vi "Main.vi"(8 "error in":errorcluster, 11 "SimulationDaq in":refnum<class "SimulationDaq.lvclass">) -> (0 "error out":errorcluster, 3 "SimulationDaq out":refnum<class "SimulationDaq.lvclass">)   [LabVIEW 2017, in "SimulationDaq.lvclass"]
doc: "The Queued Message Handler of a Worker."
uses:
  SimulationDaq.lvclass
  <vilib>/measure/NI_MABase.lvlib
  SDaqParameter.ctl
  <vilib>/addons/_Workers/Library/Classes/Message/Message.lvclass
  Initialization Data.ctl
  <vilib>/addons/_Workers/Library/Case Label.ctl
  <vilib>/addons/_Workers/Library/Workers.lvlib
  <vilib>/addons/_Workers/Library/Classes/Message Queue/Message Queue.lvclass
  <vilib>/addons/_Workers/Library/Classes/Message/Enqueue Message to Queue.vi
  <vilib>/addons/_Workers/Library/Classes/Worker/Worker.lvclass
  <vilib>/addons/_Workers/Library/Classes/Worker/Read ID.vi
  <vilib>/addons/_Workers/Library/Classes/Worker/Read Alias.vi
panel:
  out "ID out":string
  out "Alias out":string
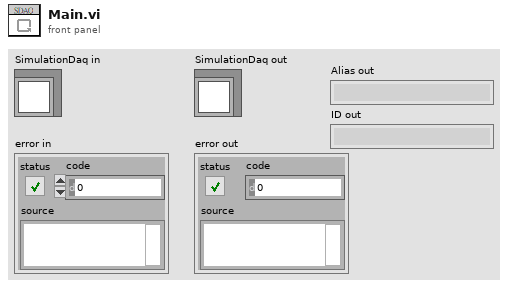
[diagram p1: front panel]
types:
  T1 = typedef "SimulationDaq.lvclass/Initialization Data.ctl" = cluster{"CallerEnQ":refnum<class "Message Queue.lvclass">, "ReturnCaseLabel":T2}
  T2 = typedef "Workers.lvlib/Case Label.ctl" = string
  T3 = typedef "SimulationDaq.lvclass/SDaqParameter.ctl" = cluster{"frequency":dbl, "amplitude":dbl, "sampling info":cluster{"Fs":dbl, "#s":dbl}}
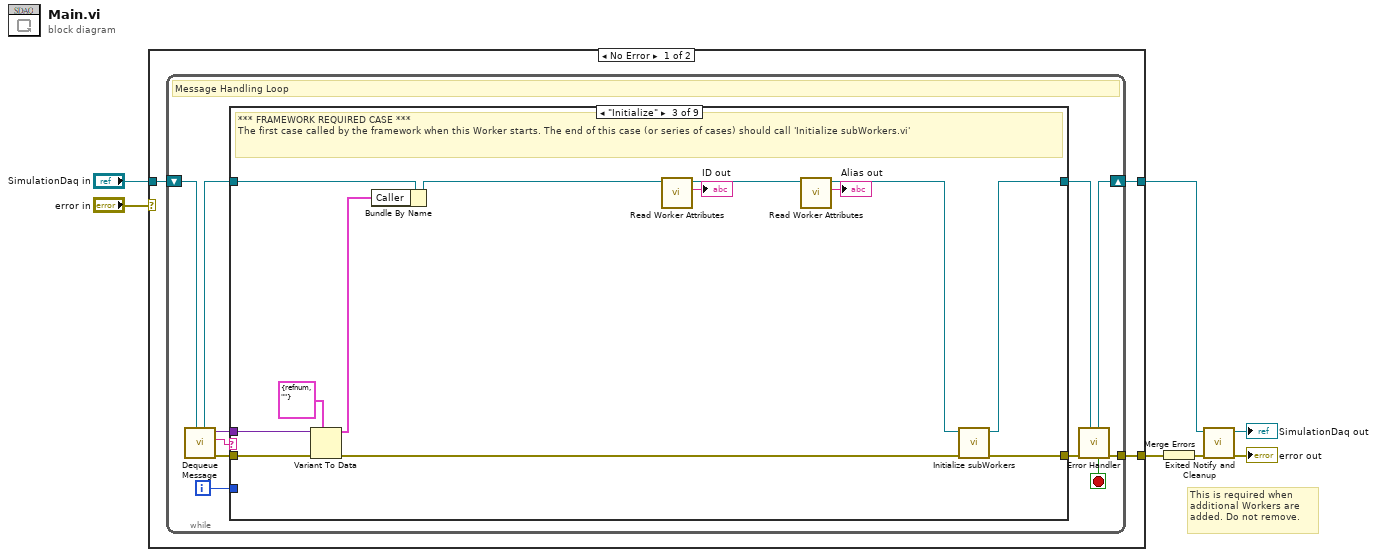
[diagram p0: block diagram]
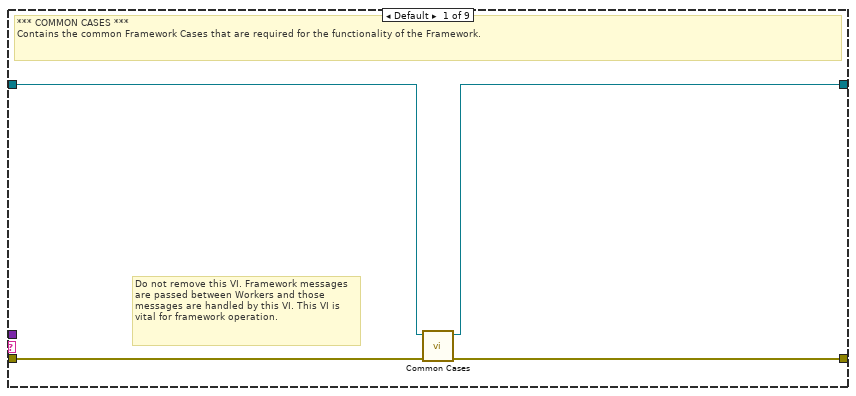
[diagram p2: hidden frame]
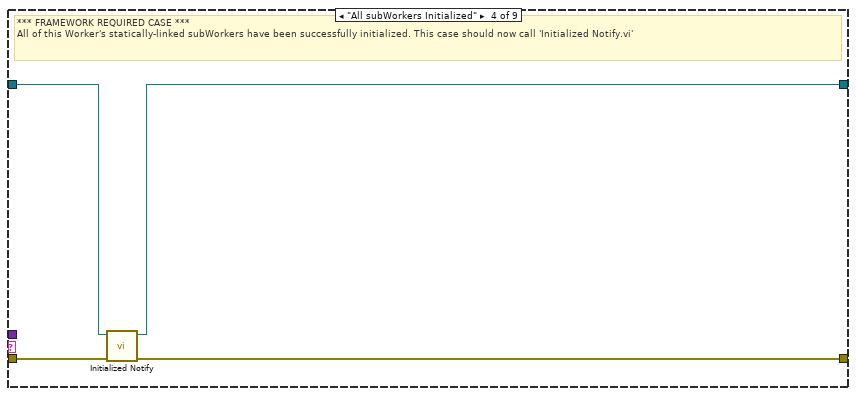
[diagram p4: hidden frame]
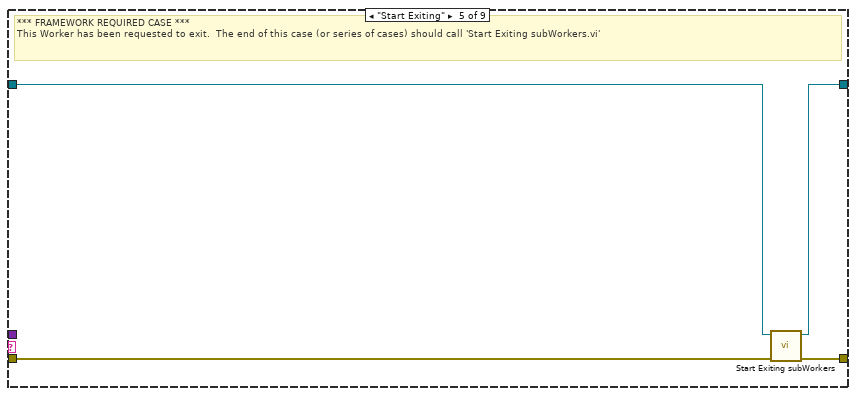
[diagram p5: hidden frame]
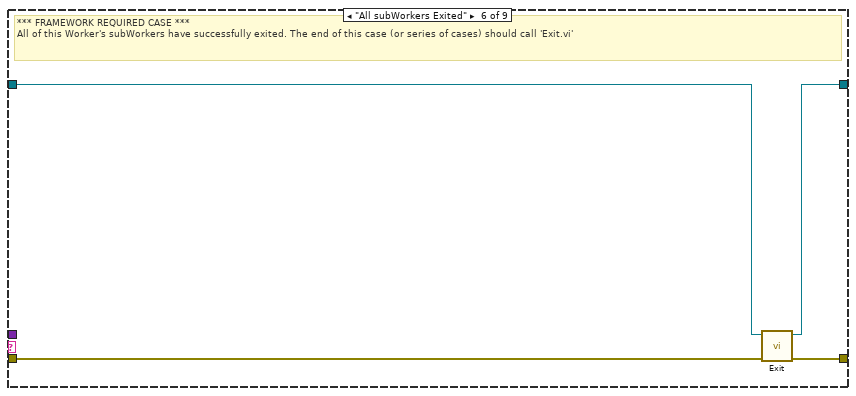
[diagram p6: hidden frame]
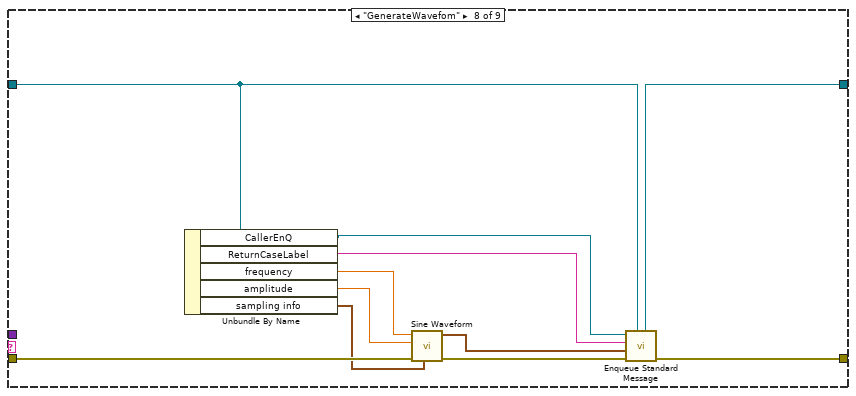
[diagram p8: hidden frame]
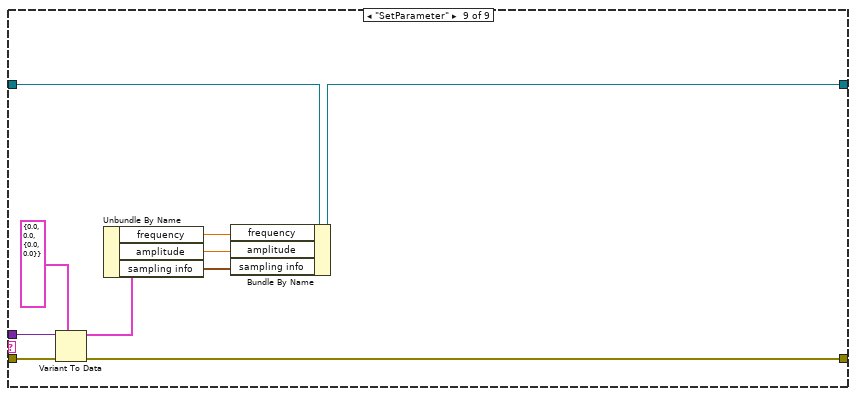
[diagram p9: hidden frame]
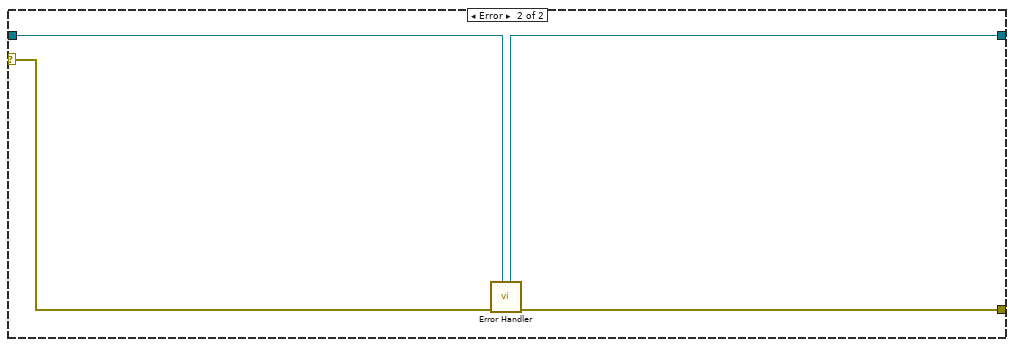
[diagram p10: hidden frame]
diagram:
  # "This is required when additional Workers are added. Do not remove."
  n1 = case shown="No Error" "error in" {
    tunnel: "SimulationDaq in" -> [w8 w77]
    tunnel: [w10 w78] -> w6
    tunnel: [w9 w76] -> w7
    selector: "error in" -> [_ w79]
    frame No Error {
      n2 = while {
        shift-right: [w19] -> w9
        shift-left: w8 -> [w21]
        tunnel: [w20] -> w10
        i -> [w11]
        stop <- w12 stop-if-true
        # "Message Handling Loop"
        n3 = call-dynamic "Dequeue Message.vi"("Worker"=w21) -> ("error out"=w18:errorcluster, "Case out"=w13:string, "Data out"=w14:variant, "Worker out"=w16:refnum<class "SimulationDaq.lvclass">)  [unwired: 6 in, 1 out]
        n4 = case "Worker MHL Case Structure (DO NOT CHANGE LABEL NAME)" shown="\"Initialize\"" w13 {
          tunnel: w18 -> [w25 w26 w38 w44 w45 w52 w53 w65 w75]
          tunnel: [w24 w26 w40 w43 w48 w51 w53 w60 w73] -> w17
          tunnel: w16 -> [w23 w27 w35 w42 w46 w50 w54 w58 w74]
          tunnel: [w22 w27 w39 w41 w47 w49 w54 w59 w70] -> w15
          tunnel: w14 -> [_ _ w36 _ _ _ _ _ w72]
          tunnel: w11 -> [_ _ _ _ _ _ _ _ _]
          frame Default {
            # "Do not remove this VI. Framework messages are passed between Workers and those messages are handled by this VI. This VI is vital for framework operation."
            # "*** COMMON CASES ***\nContains the common Framework Cases that are required for the functionality of the Framework."
            n5 = call-dynamic "Common Cases.vi"("error in"=w25, "Worker in"=w23) -> ("error out"=w24:errorcluster, "Worker out"=w22:refnum<class "SimulationDaq.lvclass">)  [unwired: 8 in]
          }
          frame "------ FRAMEWORK REQUIRED CASES ------" {
            # "Start of Framework Required Cases"
          }
          frame "Initialize" {
            # "*** FRAMEWORK REQUIRED CASE ***\nThe first case called by the framework when this Worker starts. The end of this case (or series of cases) should call 'Initialize subWorkers.vi'"
            n6 = Variant To Data(error in=w38, type=T1 {"CallerEnQ"=refnum, "ReturnCaseLabel"=""} ("Cluster"), Variant=w36) -> (data=w32:T1, error out=w37:errorcluster)
            n7 = Bundle By Name(cluster=w35, "Caller"=w32) -> (w33:refnum<class "SimulationDaq.lvclass">)
            n8 = call-poly <vilib>:"Read Worker Attributes.vi"("Worker"=w33) -> ("ID out"=→"ID out":string, "dup Worker out"=w31:refnum<class "SimulationDaq.lvclass">)  [unwired: 9 in]
            n9 = call-poly <vilib>:"Read Worker Attributes.vi"("Worker"=w31) -> ("Alias out"=→"Alias out":string, "dup Worker out"=w30:refnum<class "SimulationDaq.lvclass">)  [unwired: 9 in]
            n10 = call-dynamic "Initialize subWorkers.vi"("error in"=w37, "Worker"=w30) -> ("error out"=w40:errorcluster, "dup Worker out"=w39:refnum<class "SimulationDaq.lvclass">)  [unwired: 8 in]
          }
          frame "All subWorkers Initialized" {
            # "*** FRAMEWORK REQUIRED CASE ***\nAll of this Worker's statically-linked subWorkers have been successfully initialized. This case should now call 'Initialized Notify.vi'"
            n11 = call-dynamic "Initialized Notify.vi"("error in"=w44, "Worker"=w42) -> ("error out"=w43:errorcluster, "dup Worker out"=w41:refnum<class "SimulationDaq.lvclass">)  [unwired: 8 in]
          }
          frame "Start Exiting" {
            # "*** FRAMEWORK REQUIRED CASE ***\nThis Worker has been requested to exit.  The end of this case (or series of cases) should call 'Start Exiting subWorkers.vi'"
            n12 = call-dynamic "Start Exiting subWorkers.vi"("error_in"=w45, "Worker"=w46) -> ("error out"=w48:errorcluster, "dup Worker out"=w47:refnum<class "SimulationDaq.lvclass">)  [unwired: 8 in]
          }
          frame "All subWorkers Exited" {
            # "*** FRAMEWORK REQUIRED CASE ***\nAll of this Worker's subWorkers have successfully exited. The end of this case (or series of cases) should call 'Exit.vi'"
            n13 = call-dynamic "Exit.vi"("error_in"=w52, "Worker"=w50) -> ("error out"=w51:errorcluster, "dup Worker out"=w49:refnum<class "SimulationDaq.lvclass">)  [unwired: 8 in]
          }
          frame "-----------------------------------------------" {
            # "End of Framework Required Cases"
          }
          frame "GenerateWavefom" {
            n14 = Unbundle By Name(w58) -> ("CallerEnQ"=w57:refnum<class "Message Queue.lvclass">, "ReturnCaseLabel"=w56:T2, "frequency"=w62:dbl, "amplitude"=w61:dbl, "sampling info"=w63:cluster{"Fs":dbl, "#s":dbl})
            n15 = call <vilib>:"Sine Waveform.vi"("sampling info"=w63, "error in (no error)"=w65, "amplitude"=w61, "frequency"=w62) -> ("error out"=w64:errorcluster, "signal out"=w55:waveform(dbl))  [unwired: 6 in]
            n16 = call-poly <vilib>:"Enqueue Standard Message.vi"("Worker"=w58, "error in"=w64, "Data"=w55, "Case Label"=w56, "Message Queue"=w57) -> ("error out"=w60:errorcluster, "dup Worker out"=w59:refnum<class "SimulationDaq.lvclass">)  [unwired: 4 in, 1 out]
          }
          frame "SetParameter" {
            n17 = Variant To Data(error in=w75, type=T3 {"frequency"=0.0, "amplitude"=0.0, "sampling info"={"Fs"=0.0, "#s"=0.0}} ("SDaqParameter"), Variant=w72) -> (data=w69:T3, error out=w73:errorcluster)
            n18 = Unbundle By Name(w69) -> ("frequency"=w68:dbl, "amplitude"=w67:dbl, "sampling info"=w66:cluster{"Fs":dbl, "#s":dbl})
            n19 = Bundle By Name(cluster=w74, "frequency"=w68, "amplitude"=w67, "sampling info"=w66) -> (w70:refnum<class "SimulationDaq.lvclass">)
          }
        }
        n20 = call-dynamic "Error Handler.vi"("Worker"=w15, "error_in"=w17) -> ("error out"=w20:errorcluster, "Stop Loop"=w12:bool, "Worker out"=w19:refnum<class "SimulationDaq.lvclass">)  [unwired: 7 in]
      }
    }
    frame Error {
      n21 = call-dynamic "Error Handler.vi"("Worker"=w77, "error_in"=w79) -> ("error out"=w78:errorcluster, "Worker out"=w76:refnum<class "SimulationDaq.lvclass">)  [unwired: 7 in, 1 out]
    }
  }
  n22 = Merge Errors(w6) -> (w3:errorcluster)
  n23 = call-dynamic "Exited Notify and Cleanup.vi"("error_in"=w3, "Worker"=w7) -> ("error out"=→"error out":errorcluster, "dup Worker out"=→"SimulationDaq out":refnum<class "SimulationDaq.lvclass">)  [unwired: 8 in]
